vi "Quadrature_Encoder.vi"() -> ()   [LabVIEW 2014]
uses:
  <vilib>/rvi/Emulation/niFpgaGetClockAttributes.vi
  <vilib>/rvi/Emulation/niFpgaSctlEmulationGetInTimedLoop.vi
  <vilib>/rvi/Emulation/niFpgaEmulationReportErrorSimple.vi
  <vilib>/rvi/eio/common/nirviEmuTemplateMethod_errors.vi
  <vilib>/rvi/Emulation/niFpgaCriticalErrorInLSC.vi
  <vilib>/eio/EIONode/EIONode.xnode
panel:
  out "Position (Counts)":i16
  in  "Position Reset":bool
  in  "stop":bool
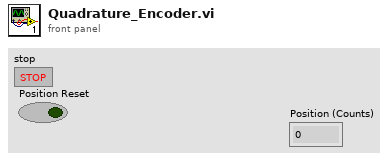
[diagram p1: front panel]
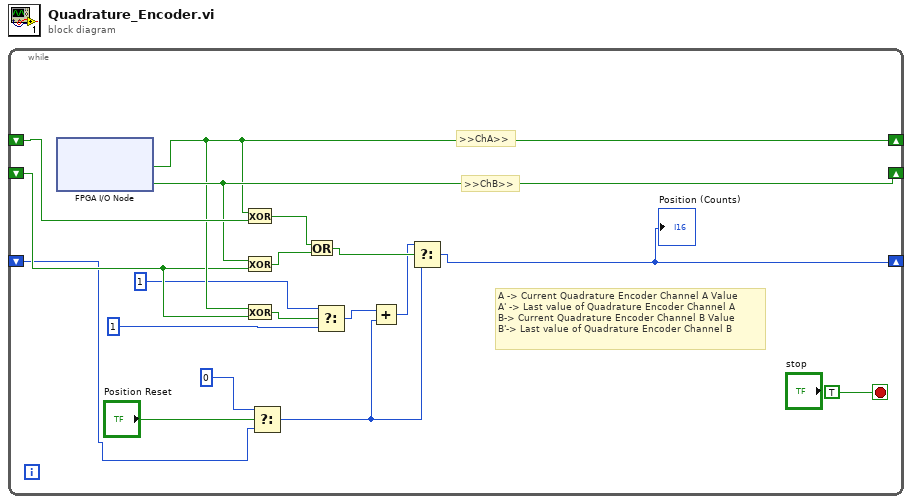
[diagram p0: block diagram]
diagram:
  n1 = while {
    shift-right: [w15] -> _
    shift-left: _ -> [w17]
    shift-right: [w16] -> _
    shift-left: _ -> [w14]
    shift-right: [w1] -> _
    shift-left: _ -> [w2]
    stop <- TRUE stop-if-true
    # "A -> Current Quadrature Encoder Channel A Value\nA' -> Last value of Quadrature Encoder Channel A\nB-> Current Quadrature Encoder Channel B Value\nB'-> Last value of Quadrature Encoder Channel B"
    # ">>ChB>>"
    # ">>ChA>>"
    n2 = xnode "FPGA I/O Node"() -> ("Mod3/DI0"=w15:bool, "Mod3/DI1"=w16:bool)  [unwired: 2 in, 2 out]
    n3 = Exclusive Or(1:w17, 2:w15) -> (0:w12:bool)
    n4 = Exclusive Or(1:w14, 2:w16) -> (0:w11:bool)
    n5 = Exclusive Or(1:w14, 2:w15) -> (0:w9:bool)
    n6 = Select(t=u32 0, s="Position Reset", f=w2) -> (s? t:f=w3:u32)
    n7 = Or(x=w12, y=w11) -> (x .or. y?=w10:bool)
    n8 = Select(t=u32 1, s=w9, f=u32 1) -> (s? t:f=w5:u32)
    n9 = Add(x=w5, y=w3) -> (x+y=w4:u32)
    n10 = Select(t=w4, s=w10, f=w3) -> (s? t:f=w1:u32)
    "Position (Counts)" <- w1
  }
